vi "GetHammerSignal.vi"(3 "column":string="hammer", 5 "Data Set":T1={"Settings"={"Data Path"=path "", "Time"=timestamp(0 s since 1904-01-01), "Sampling Rate (Hz)"=44800, "Device"=0, "pre-trigger (sec)"=100.0, "length of sample (sec)"=1000.0, "trigger value (V)"=100.0, "Labels"=[], "Cutoffs (sec)"=[], "Freq Bands"=[]}, "Data"=[], "Plot type"=enum."Linear"} {"Settings"."Time" format="%<%H:%M\n%d/%m/%y>T"}) -> (0 "Cutoff":dbl, 1 "Data set":dbl[](array[numeric]), 2 "time between samples":dbl)   [LabVIEW 2014]
uses:
  <userlib>/CurtinCode/DataControl.ctl
  <userlib>/CurtinCode/SettingsControl.ctl
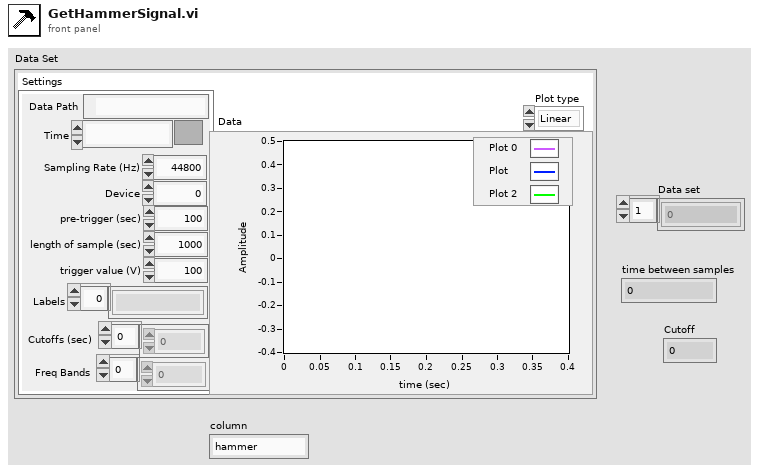
[diagram p1: front panel]
types:
  T1 = typedef "DataControl.ctl" = cluster{"Settings":T2, "Data":cluster{i32, dbl, "data":dbl[]}[], "Plot type":enum16{"Linear", "log"}}
  T2 = typedef "SettingsControl.ctl" = cluster{"Data Path":path, "Time":timestamp, "Sampling Rate (Hz)":u16, "Device":u16, "pre-trigger (sec)":dbl, "length of sample (sec)":dbl, "trigger value (V)":dbl, "Labels":string[], "Cutoffs (sec)":dbl[], "Freq Bands":dbl[]}
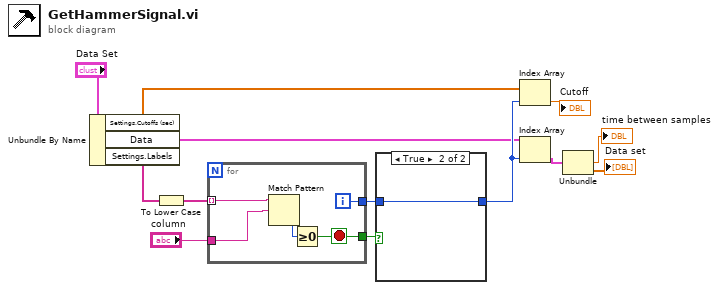
[diagram p0: block diagram]
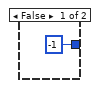
[diagram p2: hidden frame]
diagram:
  n1 = Unbundle By Name("Data Set") -> ("Settings.Cutoffs (sec)"=w7:dbl[], "Data"=w4:cluster{i32, dbl, "data":dbl[]}[], "Settings.Labels"=w8:string[])
  n2 = To Lower Case(string=w8) -> (all lower case string=w11:string[])
  n3 = for {
    tunnel: w11 -> [w18] mode=indexing
    tunnel: [w16] -> w12
    tunnel: [w15] -> w13
    tunnel: "column" -> [w14]
    i -> [w15]
    stop <- w16 stop-if-true
    n4 = Match Pattern(string=w18, regular expression=w14) -> (offset past match=w17:i32)  [unwired: 1 in, 3 out]
    n5 = Greater Or Equal To 0?(x=w17) -> (x >= 0?=w16:bool)
  }
  n6 = case shown="True" w12 {
    tunnel: w13 -> [_ w20]
    tunnel: [-1 w20] -> w5
    frame False {
    }
    frame True {
    }
  }
  n7 = Index Array(array=w7, index=w5) -> (element=→"Cutoff":dbl)
  n8 = Index Array(array=w4, index=w5) -> (element=w3:cluster{i32, dbl, "data":dbl[]})
  n9 = Unbundle(w3) -> (→"time between samples":dbl, "data"=→"Data set":dbl[])  [unwired: 1 out]
